vi "_066.vi"   [LabVIEW 2024]
panel:
  # "Mouse Coursor :"
  # "How to change your mouse coursor to busy state when an operation is going on ?"
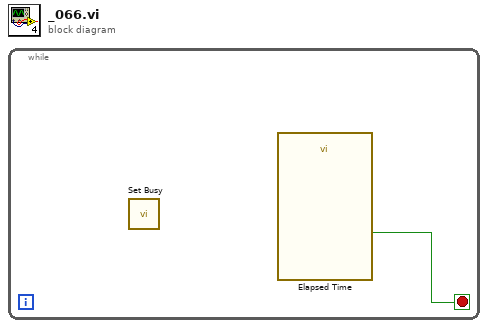
[diagram p0: block diagram]
diagram:
  n1 = while {
    stop <- w1 stop-if-true
    n2 = call <vilib>:"Set Busy.vi"() -> ()  [unwired: 10 in, 2 out]
    n3 = call "Elapsed Time"() -> ("Time has Elapsed"=w1:bool)  [unwired: 12 in, 7 out]
  }
